vi "My Nonlinear Curve Fit LM bounds.vi"(0 "Y":dbl[](array[numeric]), 1 "f(x,a)":T5, 2 "data":variant, 5 "X":dbl[](array[numeric]), 7 "Weight":dbl[](array[numeric]), 9 "initial parameters":dbl[](array[numeric]), 11 "error in (no error)":errorcluster, 12 "Termination Criteria":T6={"Max Iterations"=1000, "Max Function Calls"=10000, "Max Time"=1000.0, "Function Tolerance"=1e-06, "Parameter Tolerance"=1e-06, "Gradient Tolerance"=1e-06, "Min Lambda"=1e-06, "Max Lambda"=1000000.0, "Initial Tick Count"=0}, 13 "parameter bounds":T3, 14 "NL Fit Method":T4) -> (3 "Fit Aborted?":bool, 4 "best nonlinear fit":dbl[](array[numeric]), 6 "best fit parameters":dbl[](array[numeric]), 8 "covariance":T7, 10 "Fit Statistics":T1={"# Iterations"=0, "# Function Calls"=0, "Chi2"=0.0, "Chi2/DOF"=0.0, "Fit Convergence Criterion"=enum."Continue", "Gradient"=0.0, "|Delta Chi 2|"=0.0, "|Delta Chi 2|/Chi 2"=0.0, "Max |Delta a| /|a|"=0.0, "Lambda"=-1.0, "Weighted Chi2"=-1.0, "Unweighted Chi2"=-1.0}, 15 "error out":errorcluster)   [LabVIEW 2021, in "Fits.lvlib"]
uses:
  Fits.lvlib
  <vilib>/Analysis/Matrix/Datatypes/RealMatrix.ctl
  My Fit Stopping Criteria.ctl
  <vilib>/gmath/NumericalOptimization/LM model function reference.ctl
  Nonlinear Fit Method.ctl
  Fit Statistics v3.ctl
  Convergence Criteria.ctl
  <vilib>/gmath/NumericalOptimization/LM model function.ctl
  <userlib>/_OpenG.lib/array/array.llb/Remove Duplicates from 1D Array (DBL)__ogtk.vi
  Abort Fit Global.vi
  <vilib>/Analysis/baseanly.llb/Real Inverse Matrix.vi
  <vilib>/gmath/NumericalOptimization/LM_output select.ctl
  <vilib>/gmath/NI_Gmath.lvlib
  <vilib>/Analysis/NI_AALBase.lvlib
  <userlib>/_OpenG.lib/array/array.llb/openg_array.lvlib
  <vilib>/Analysis/Matrix/NI_Matrix.lvlib
panel:
  out "Lambda Chart":dbl(graph)
  out "Parameters Gradient Chart":dbl[][](graph)
  in  "Repeat Fit N times (1)":i32=1
  in  "Reset Charts":bool
  out "Chi2 Chart":dbl(graph)
  out "Parameters Graph":dbl[](graph)
  in  "Delay (ms)":i32
  in  "Debug":bool
  out "Parameters Chart":dbl[][](graph)
  out "Function & Fit Graph":cluster{"New Coefficients":dbl[]}[](graph)
  # "see the AlliGator License on the block diagram (Ctrl+E or Window:Show Block Diagram)"
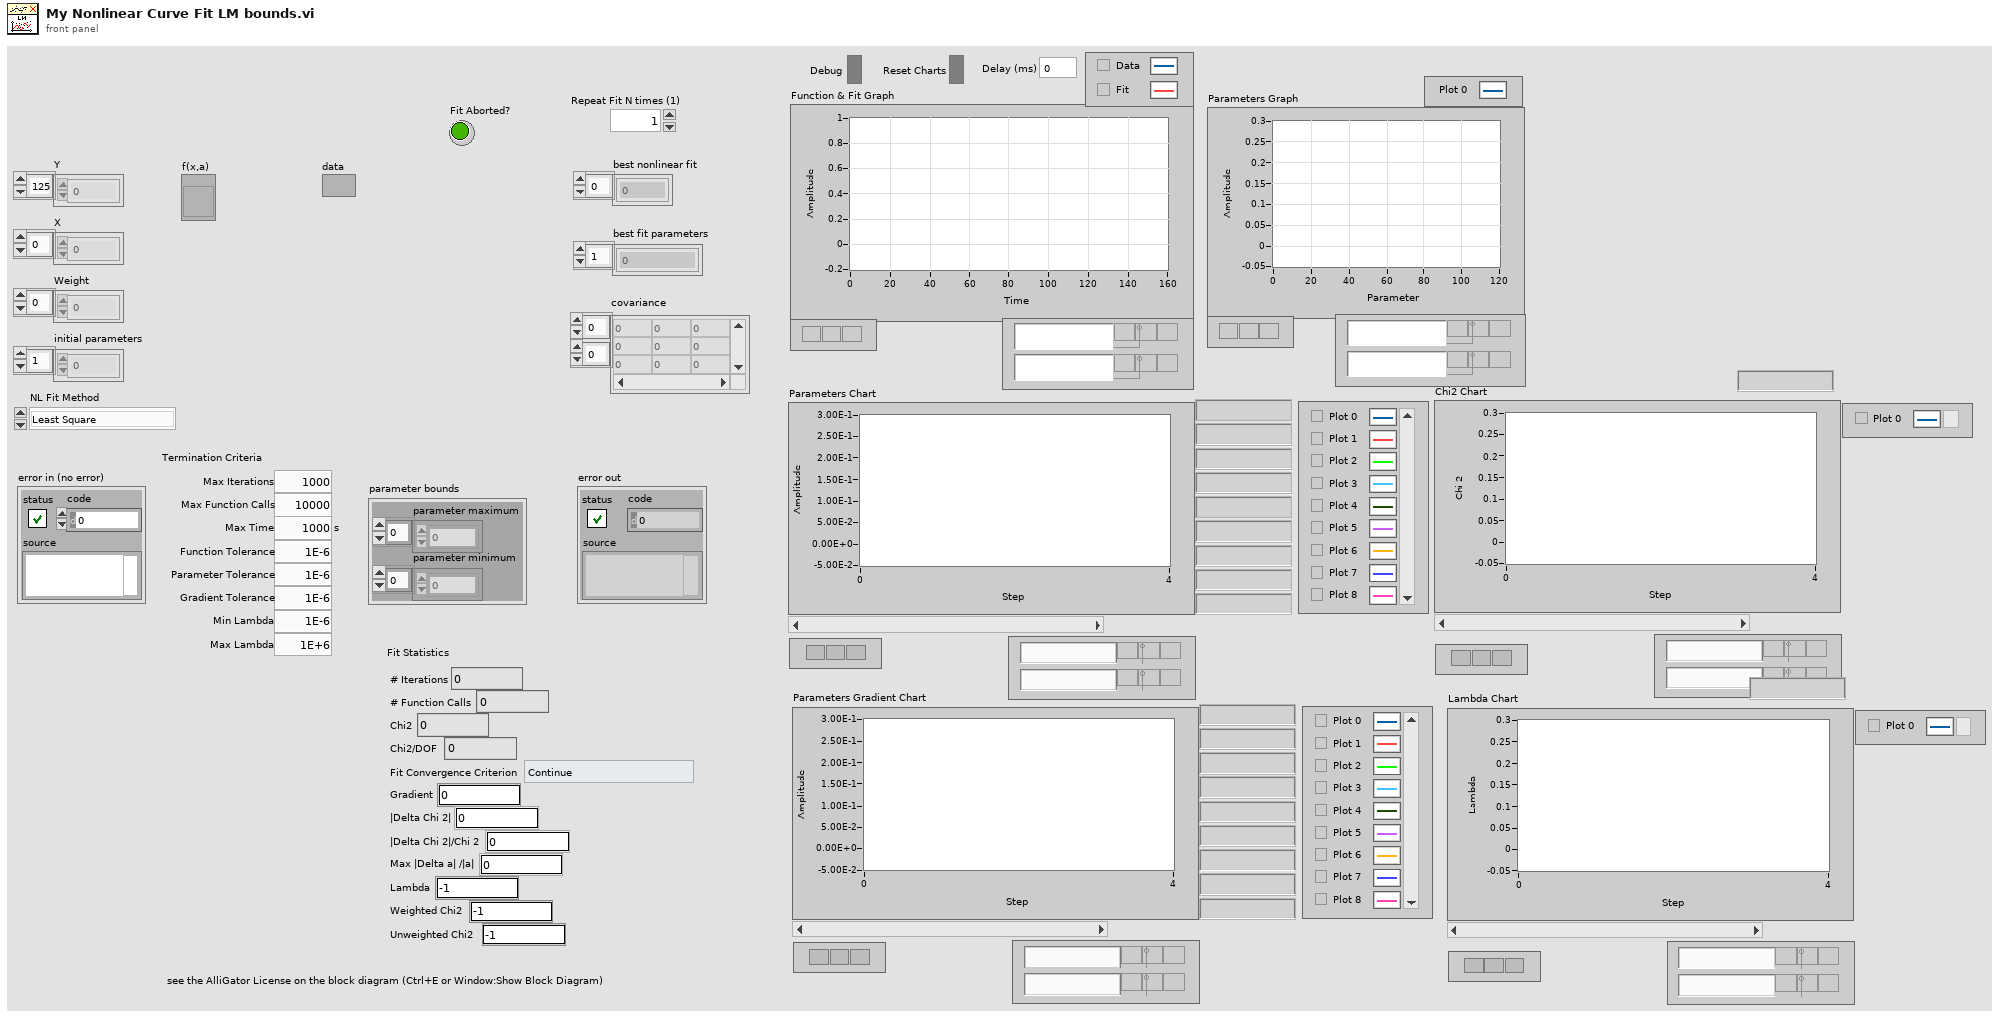
[diagram p1: front panel]
types:
  T1 = typedef "Fits.lvlib/Fit Statistics v3.ctl" = cluster{"# Iterations":i32, "# Function Calls":i32, "Chi2":dbl, "Chi2/DOF":dbl, "Fit Convergence Criterion":T2, "Gradient":dbl, "|Delta Chi 2|":dbl, "|Delta Chi 2|/Chi 2":dbl, "Max |Delta a| /|a|":dbl, "Lambda":dbl, "Weighted Chi2":dbl, "Unweighted Chi2":dbl}
  T2 = typedef "Fits.lvlib/Convergence Criteria.ctl" = enum16{"Continue", "Tolerances Exceeded", "Max Time Exceeded", "Max Iterations Exceeded", "Max Function Evaluations Exceeded", "Scale Range Exceeded"}
  T3 = cluster{"parameter minimum":dbl[], "parameter maximum":dbl[]}
  T4 = typedef "Fits.lvlib/Nonlinear Fit Method.ctl" = enum16{"Least Square", "Least Absolute Residual", "Bisquare", "MLE"}
  T5 = typedef "NI_Gmath.lvlib/LM model function reference.ctl" = refnum<vi>
  T6 = typedef "Fits.lvlib/My Fit Stopping Criteria.ctl" = cluster{"Max Iterations":i32, "Max Function Calls":i32, "Max Time":dbl[unit], "Function Tolerance":dbl, "Parameter Tolerance":dbl, "Gradient Tolerance":dbl, "Min Lambda":dbl, "Max Lambda":dbl, "Initial Tick Count":u32}
  T7 = typedef "NI_Matrix.lvlib/RealMatrix.ctl" = dbl[][]
  T8 = typedef "NI_Gmath.lvlib/LM model function.ctl" = cluster{"f(x,a)":T5, "data":variant}
  T9 = typedef "NI_Gmath.lvlib/LM_output select.ctl" = cluster{"model function":bool, "gradient":bool}
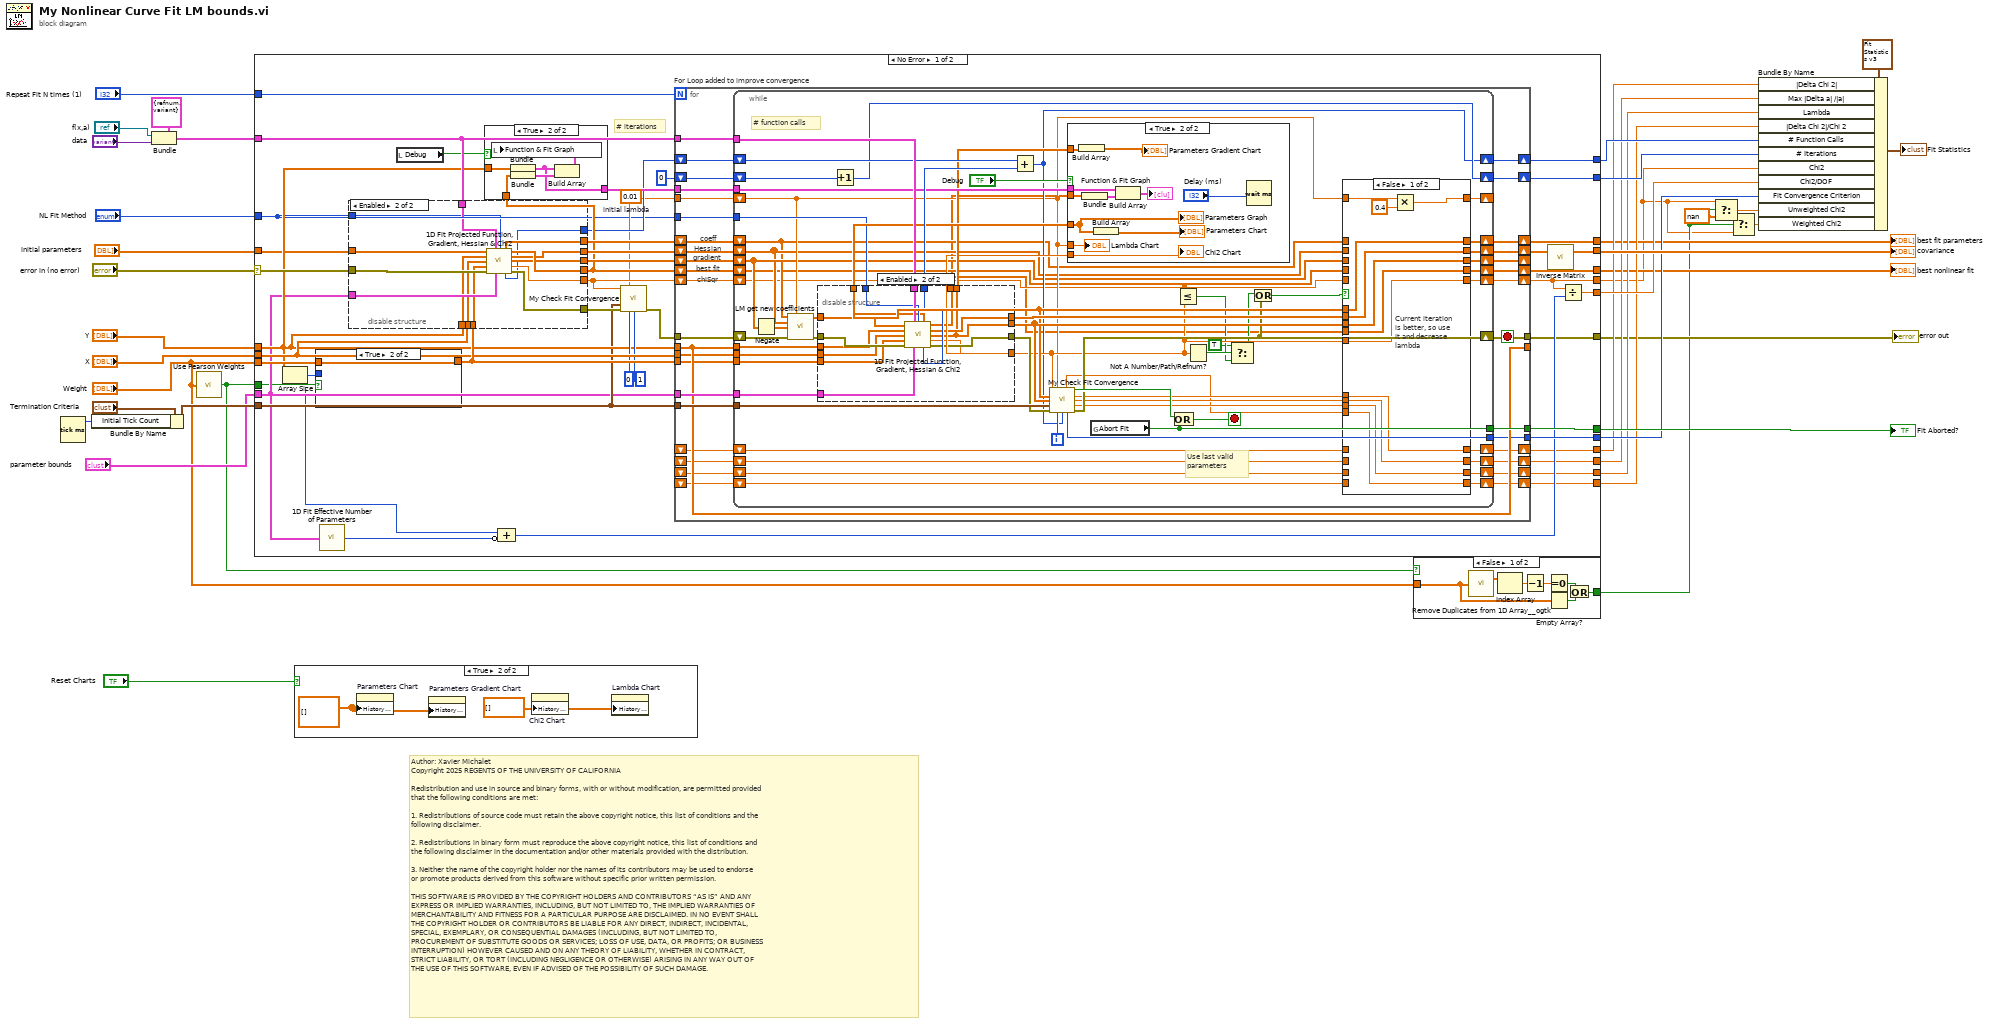
[diagram p0: block diagram]
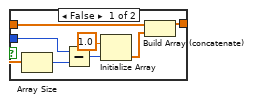
[diagram p3: hidden frame]
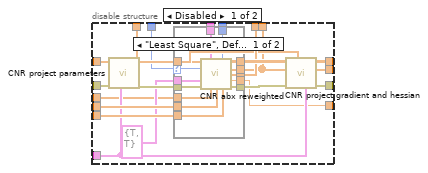
[diagram p4: hidden frame]
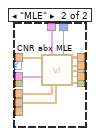
[diagram p5: hidden frame]
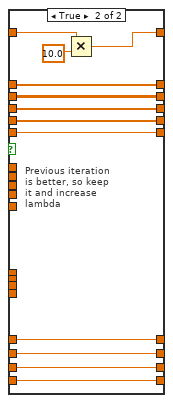
[diagram p7: hidden frame]
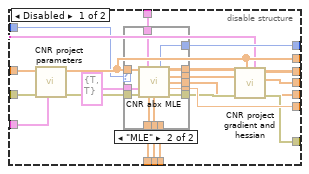
[diagram p8: hidden frame]
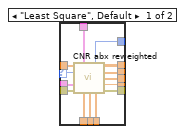
[diagram p9: hidden frame]
diagram:
  w9 = nan ("f")
  # "Author: Xavier Michalet\nCopyright 2025 REGENTS OF THE UNIVERSITY OF CALIFORNIA\n\nRedistribution and use in source and binary forms, with or without modification, are permitted provided\nthat the following conditions are met:\n\n1. Redistributions of source code must retain the above copyright notice, this list of conditions and the\nfollowing disclaimer.\n\n2. Redistributions in binary form must reproduce the above copyright notice, this list of conditions and\nthe following disclaimer in the documentation and/or other materials provided with the distribution.\n\n3. Neither the name of the copyright holder nor the names of its contributors may be used to endorse \nor promote products derived from this software without specific prior written permission.\n\nTHIS SOFTWARE IS PROVIDED BY THE COPYRIGHT HOLDERS AND CONTRIBUTORS “AS IS” AND ANY \nEXPRESS OR IMPLIED WARRANTIES, INCLUDING, BUT NOT LIMITED TO, THE IMPLIED WARRANTIES OF\nMERCHANTABILITY AND FITNESS FOR A PARTICULAR PURPOSE ARE DISCLAIMED. IN NO EVENT SHALL\nTHE COPYRIGHT HOLDER OR CONTRIBUTORS BE LIABLE FOR ANY DIRECT, INDIRECT, INCIDENTAL, \nSPECIAL, EXEMPLARY, OR CONSEQUENTIAL DAMAGES (INCLUDING, BUT NOT LIMITED TO, \nPROCUREMENT OF SUBSTITUTE GOODS OR SERVICES; LOSS OF USE, DATA, OR PROFITS; OR BUSINESS\nINTERRUPTION) HOWEVER CAUSED AND ON ANY THEORY OF LIABILITY, WHETHER IN CONTRACT, \nSTRICT LIABILITY, OR TORT (INCLUDING NEGLIGENCE OR OTHERWISE) ARISING IN ANY WAY OUT OF\nTHE USE OF THIS SOFTWARE, EVEN IF ADVISED OF THE POSSIBILITY OF SUCH DAMAGE."
  n1 = Tick Count (ms)() -> (millisecond timer value=w25:u32)
  n2 = Bundle By Name(cluster="Termination Criteria", "Initial Tick Count"=w25) -> (w24:T6)
  n3 = Bundle(cluster=T8 {"f(x,a)"=refnum, "data"=variant} ("model function"), "f(x,a)"="f(x,a)", "data"="data") -> (w15:T8)
  n4 = call "Use Pearson Weights.vi"("Weight"="Weight") -> ("Use Pearson Weight"=w1:bool)
  n5 = case shown="No Error" "error in (no error)" {
    selector: "error in (no error)" -> [w66 w346]
    tunnel: [w67 _] -> w13
    tunnel: [w80 _] -> w27
    tunnel: "initial parameters" -> [w48 _]
    tunnel: [w73 _] -> w6
    tunnel: [w79 _] -> w36
    tunnel: "Weight" -> [w78 _]
    tunnel: "Y" -> [w60 _]
    tunnel: w24 -> [w53 _]
    tunnel: "X" -> [w74 _]
    tunnel: [w45 w346] -> w5
    tunnel: w15 -> [w75 _]
    tunnel: [w68 _] -> w30
    tunnel: "NL Fit Method" -> [w44 _]
    tunnel: "parameter bounds" -> [w47 _]
    tunnel: [w61 _] -> w31
    tunnel: [w56 _] -> w3
    tunnel: [w54 _] -> w28
    tunnel: "Repeat Fit N times (1)" -> [w51 _]
    tunnel: [w50 _] -> w20
    tunnel: [w43 _] -> w17
    tunnel: [w42 _] -> w19
    tunnel: [w41 _] -> w18
    tunnel: [w40 _] -> w16
    tunnel: w1 -> [w39 _]
    frame No Error {
      w52 = 0.01  # initial lambda
      # "# iterations"
      n6 = Array Size(array=w60) -> (size(s)=w38:i32)
      n7 = case shown="True" w39 {
        tunnel: [w88 w89] -> w81
        tunnel: w78 -> [w83 w89]
        tunnel: w38 -> [w82 _]
        frame False {
          n8 = Array Size(array=w83) -> (size(s)=w86:i32)
          n9 = Subtract(x=w82, y=w86) -> (x-y=w85:i32)
          n10 = Initialize Array(1.0, w85) -> (w84:dbl[])
          n11 = Build Array (concatenate)(w83, w84) -> (w88:dbl[])
        }
        frame True {
        }
      }
      n12 = call "1D Fit Effective Number of Parameters.vi"("parameter bounds"=w47) -> ("Effective Number of Parameters"=w46:i32)  [unwired: 8 in]
      n13 = disable-structure shown="Enabled" {
        disable-tunnel: w81 -> [w299 w329]
        disable-tunnel: [w298 w337] -> w77
        disable-tunnel: w75 -> [w297 w340]
        disable-tunnel: w74 -> [w296 w328]
        disable-tunnel: w66 -> [w294 w330]
        disable-tunnel: [w291 w336] -> w65
        disable-tunnel: [w288 w339] -> w64
        disable-tunnel: [w287 w335] -> w63
        disable-tunnel: [w286 w334] -> w62
        disable-tunnel: w60 -> [w285 w327]
        disable-tunnel: [w284 w338] -> w58
        disable-tunnel: [w283 w333] -> w55
        disable-tunnel: w48 -> [w282 w326]
        disable-tunnel: w47 -> [w281 w331]
        disable-tunnel: w44 -> [w280 w332]
        frame Disabled {
          n14 = call <vilib>:"CNR project parameters.vi"("bounds"=w281, "error in"=w294, "parameters"=w282) -> ("error out"=w293:errorcluster, "projected parameters"=w288:dbl[])  [unwired: 7 out]
          n15 = case shown="\"MLE\"" w280 {
            selector: w280 -> [w303 _]
            tunnel: w299 -> [w313 _]
            tunnel: [w312 w318] -> w298
            tunnel: w297 -> [w311 w325]
            tunnel: w296 -> [w310 w319]
            tunnel: T9 {"model function"=TRUE, "gradient"=TRUE} ("output control") -> [w309 w323]
            tunnel: w293 -> [w308 w322]
            tunnel: [w307 w321] -> w292
            tunnel: [w306 w315] -> w290
            tunnel: [w305 w316] -> w289
            tunnel: w288 -> [w304 w324]
            tunnel: w285 -> [w302 w320]
            tunnel: [w301 w317] -> w284
            tunnel: [w300 w314] -> w283
            frame "Least Square", Default {
              n16 = call <vilib>:"CNR abx reweighted.vi"("parameters"=w304, "model function"=w311, "method"=w303, "output control"=w309, "error in (no error)"=w308, "Y"=w302, "X"=w310, "Weight"=w313) -> ("number of function calls"=w300:i32, "Hessian"=w306:T7, "gradient"=w305:dbl[], "best fit"=w301:dbl[], "chiSqr"=w312:dbl, "error out"=w307:errorcluster)  [unwired: 1 in, 1 out]
            }
            frame "MLE" {
              n17 = call "CNR abx MLE.vi"("parameters"=w324, "model function"=w325, "output control"=w323, "error in (no error)"=w322, "Y"=w320, "X"=w319) -> ("number of function calls"=w314:i32, "Hessian"=w315:T7, "gradient"=w316:dbl[], "best fit"=w317:dbl[], "chiSqr"=w318:dbl, "error out"=w321:errorcluster)  [unwired: 3 in, 1 out]
            }
          }
          n18 = call <vilib>:"CNR project gradient and hessian.vi"("bounds"=w281, "projected parameters"=w288, "error in"=w292, "gradient"=w289, "Hessian"=w290) -> ("error out"=w291:errorcluster, "projected gradient"=w286:dbl[], "projected Hessian"=w287:T7)  [unwired: 1 in, 3 out]
        }
        frame Enabled {
          n19 = call "1D Fit Projected Function, Gradient, Hessian & Chi2.vi"("parameters"=w326, "model function"=w340, "NL Fit Method"=w332, "Y"=w327, "X"=w328, "Weights"=w329, "Error In"=w330, "Parameter Bounds"=w331) -> ("projected parameters"=w339:dbl[], "best fit"=w338:dbl[], "projected Hessian"=w335:T7, "projected gradient"=w334:dbl[], "Chi2"=w337:dbl, "number of function calls"=w333:i32, "Error Out"=w336:errorcluster)  [unwired: 1 in]
        }
      }
      n20 = local read "Debug"() -> (w57:bool)
      n21 = case shown="True" w57 {
        tunnel: w60 -> [_ w345]
        tunnel: [_ w342] -> w59
        tunnel: w58 -> [_ w344]
        frame False {
        }
        frame True {
          n22 = Bundle("Y"=w345) -> (w342:cluster{"Y":dbl[]})  [unwired: 1 in]
          n23 = Bundle("best fit"=w344) -> (w343:cluster{"best fit":dbl[]})  [unwired: 1 in]
          n24 = Build Array(w342, w343) -> (w341:cluster{"best fit":dbl[]}[])
          n25 = local write "Function & Fit Graph"(w341) -> ()
        }
      }
      n26 = Compound Arithmetic op=ADD(w38, invert w46) -> (w49:i32)
      n27 = call "My Check Fit Convergence.vi"("Chi 2"=w77, "Lambda"=w52, "my stopping criteria"=w53, "Error In"=w65, "current iteration"=0, "number of function evaluations"=1) -> ("error out"=w76:errorcluster)  [unwired: 2 in, 7 out]
      n28 = for "For Loop added to improve convergence" {
        N: w51 -> [_]
        tunnel: w75 -> [w122]
        tunnel: w47 -> [w115]
        tunnel: w44 -> [w112]
        tunnel: [w111] -> w61
        tunnel: w59 -> [w110]
        tunnel: w53 -> [w105]
        shift-right: [w108] -> w56
        shift-left: w77 -> [w124]
        shift-right: [w118] -> w68
        shift-left: w55 -> [w107]
        shift-right: [w106] -> w54
        shift-left: 0 -> [w119]
        tunnel: w52 -> [w104]
        shift-right: [w117] -> w67
        shift-left: w64 -> [w116]
        shift-right: [w120] -> w70
        shift-left: w63 -> [w114]
        shift-right: [w103] -> _
        shift-left: w62 -> [w113]
        shift-right: [w121] -> w73
        shift-left: w58 -> [w109]
        tunnel: [w99] -> w50
        tunnel: w76 -> [w123]
        tunnel: [w98] -> w45
        shift-right: [w96] -> w42
        shift-left: _ -> [w92]
        shift-right: [w97] -> w43
        shift-left: _ -> [w91]
        shift-right: [w95] -> w41
        shift-left: _ -> [w93]
        shift-right: [w94] -> w40
        shift-left: _ -> [w90]
        tunnel: w81 -> [w100]
        tunnel: w74 -> [w101]
        tunnel: w60 -> [w102]
        tunnel: [w102] -> _
        stop <- w98 stop-if-true
        # "best fit"
        # "chiSqr"
        # "gradient"
        # "Hessian"
        # "coeff"
        n29 = while {
          tunnel: w101 -> [w179]
          tunnel: w102 -> [w161]
          tunnel: w100 -> [w178]
          shift-left: w124 -> [w126]
          shift-right: [w170] -> w108
          shift-left: w113 -> [w130]
          shift-right: [w182] -> w103
          shift-left: w114 -> [w129]
          shift-right: [w183] -> w120
          shift-left: w116 -> [w128]
          shift-right: [w171] -> w117
          shift-left: w104 -> [w131]
          shift-right: [w180] -> _
          shift-right: [w152] -> w98
          shift-left: w123 -> [w181]
          tunnel: w122 -> [w177]
          tunnel: w105 -> [w173]
          shift-right: [w132] -> w118
          shift-left: w107 -> [w176]
          shift-right: [w175] -> w121
          shift-left: w109 -> [w127]
          shift-right: [w133] -> w106
          shift-left: w119 -> [w158]
          tunnel: w112 -> [w146]
          tunnel: w115 -> [w166]
          tunnel: [w163] -> w111
          tunnel: w110 -> [w160]
          tunnel: [w154] -> w99
          shift-right: [w141] -> w95
          shift-left: w93 -> [w137]
          shift-right: [w140] -> w96
          shift-left: w92 -> [w136]
          shift-right: [w139] -> w97
          shift-left: w91 -> [w135]
          shift-right: [w138] -> w94
          shift-left: w90 -> [w134]
          i -> [w157]
          stop <- w156 stop-if-true
          # "# function calls"
          # "Use last valid parameters"
          n30 = Negate(x=w130) -> (-x=w164:dbl[])
          n31 = call <vilib>:"LM get new coefficients.vi"("Coefficients"=w128, "lamda"=w131, "Alpha"=w129, "Beta"=w164, "error in (no error)"=w181) -> ("New Coefficients"=w162:dbl[], "error out"=w169:errorcluster)  [unwired: 9 out]
          n32 = disable-structure shown="Enabled" {
            disable-tunnel: [w204 w243] -> w184
            disable-tunnel: w179 -> [w203 w231]
            disable-tunnel: w178 -> [w202 w230]
            disable-tunnel: w177 -> [w201 w244]
            disable-tunnel: w169 -> [w200 w241]
            disable-tunnel: [w197 w242] -> w168
            disable-tunnel: [w196 w235] -> w167
            disable-tunnel: w166 -> [w195 w240]
            disable-tunnel: [w193 w237] -> w165
            disable-tunnel: w162 -> [w191 w239]
            disable-tunnel: w161 -> [w190 w232]
            disable-tunnel: [w189 w236] -> w125
            disable-tunnel: [w188 w233] -> w155
            disable-tunnel: [w187 w235] -> w153
            disable-tunnel: [w186 w238] -> w151
            disable-tunnel: w146 -> [w185 w234]
            frame Disabled {
              n33 = call <vilib>:"CNR project parameters.vi"("bounds"=w195, "error in"=w200, "parameters"=w191) -> ("error out"=w199:errorcluster, "projected parameters"=w188:dbl[])  [unwired: 7 out]
              n34 = case shown="\"Least Square\", Default" w185 {
                selector: w185 -> [w210 _]
                tunnel: [w218 w224] -> w204
                tunnel: w203 -> [w217 w225]
                tunnel: w202 -> [w216 _]
                tunnel: w201 -> [w215 w228]
                tunnel: w199 -> [w214 _]
                tunnel: [w213 w219] -> w198
                tunnel: [w212 w223] -> w194
                tunnel: T9 {"model function"=TRUE, "gradient"=TRUE} ("output control") -> [w211 w227]
                tunnel: w190 -> [w209 w226]
                tunnel: [w208 w221] -> w189
                tunnel: w188 -> [w207 w229]
                tunnel: [w206 w222] -> w187
                tunnel: [w205 w220] -> w186
                frame "Least Square", Default {
                  n35 = call <vilib>:"CNR abx reweighted.vi"("parameters"=w207, "model function"=w215, "method"=w210, "output control"=w211, "error in (no error)"=w214, "Y"=w209, "X"=w217, "Weight"=w216) -> ("number of function calls"=w218:i32, "Hessian"=w212:T7, "gradient"=w206:dbl[], "best fit"=w208:dbl[], "chiSqr"=w205:dbl, "error out"=w213:errorcluster)  [unwired: 1 in, 1 out]
                }
                frame "MLE" {
                  n36 = call "CNR abx MLE.vi"("parameters"=w229, "model function"=w228, "output control"=w227, "Y"=w226, "X"=w225) -> ("number of function calls"=w224:i32, "Hessian"=w223:T7, "gradient"=w222:dbl[], "best fit"=w221:dbl[], "chiSqr"=w220:dbl, "error out"=w219:errorcluster)  [unwired: 4 in, 1 out]
                }
              }
              n37 = call <vilib>:"CNR project gradient and hessian.vi"("bounds"=w195, "projected parameters"=w188, "error in"=w198, "gradient"=w187, "Hessian"=w194) -> ("error out"=w197:errorcluster, "projected gradient"=w196:dbl[], "projected Hessian"=w193:T7)  [unwired: 1 in, 3 out]
            }
            frame Enabled {
              n38 = call "1D Fit Projected Function, Gradient, Hessian & Chi2.vi"("parameters"=w239, "model function"=w244, "NL Fit Method"=w234, "Y"=w232, "X"=w231, "Weights"=w230, "Error In"=w241, "Parameter Bounds"=w240) -> ("projected parameters"=w233:dbl[], "best fit"=w236:dbl[], "projected Hessian"=w237:T7, "projected gradient"=w235:dbl[], "Chi2"=w238:dbl, "number of function calls"=w243:i32, "Error Out"=w242:errorcluster)  [unwired: 1 in]
            }
          }
          n39 = Increment(x=w158) -> (x+1=w133:i32)
          n40 = Add(x=w176, y=w184) -> (x+y=w132:i32)
          n41 = call "My Check Fit Convergence.vi"("Chi 2"=w151, "Lambda"=w131, "Parameters"=w155, "gradient"=w167, "my stopping criteria"=w173, "Error In"=w168, "current iteration"=w157, "number of function evaluations"=w132) -> ("|Delta Chi 2|/Chi 2"=w142:dbl, "stop?"=w172:bool, "|Delta Chi 2|"=w145:dbl, "Max |Delta a| /|a|"=w144:dbl, "Lambda"=w143:dbl, "Convergence Criterium Reached"=w154:T2, "error out"=w152:errorcluster)  [unwired: 1 out]
          n42 = case shown="True" "Debug" {
            tunnel: w155 -> [_ w248]
            tunnel: w160 -> [_ w255]
            tunnel: w125 -> [_ w252]
            tunnel: w151 -> [_ w250]
            tunnel: w153 -> [_ w249]
            tunnel: w131 -> [_ w245]
            frame False {
            }
            frame True {
              n43 = Build Array(w249) -> (→"Parameters Gradient Chart":dbl[][])
              n44 = Bundle("best fit"=w252) -> (w254:cluster{"best fit":dbl[]})  [unwired: 1 in]
              n45 = Build Array(w248) -> (→"Parameters Chart":dbl[][])
              n46 = Build Array(w255, w254) -> (→"Function & Fit Graph":cluster{"best fit":dbl[]}[])
              n47 = Wait (ms)(milliseconds to wait="Delay (ms)") -> ()  [unwired: 1 out]
              "Parameters Graph" <- w248
              "Chi2 Chart" <- w250
              "Lambda Chart" <- w245
            }
          }
          n48 = global read "Abort Fit Global.vi" "Abort Fit"() -> (w163:bool)
          n49 = Compound Arithmetic op=OR(w172, w163) -> (w156:bool)
          n50 = Less Or Equal?(x=w126, y=w151) -> (x <= y?=w149:bool)
          n51 = Not A Number/Path/Refnum?(number/path/refnum=w151) -> (NaN/Path/Refnum?=w150:bool)
          n52 = Select(t=TRUE, s=w150, f=w149) -> (s? t:f=w147:bool)
          n53 = Or(x=w147, y=w152) -> (x .or. y?=w174:bool)
          n54 = case shown="False" w174 {
            tunnel: [w266 w279] -> w183
            tunnel: w129 -> [_ w279]
            tunnel: [w265 w278] -> w182
            tunnel: w155 -> [w262 _]
            tunnel: w130 -> [_ w278]
            tunnel: w128 -> [_ w277]
            tunnel: [w262 w277] -> w171
            tunnel: [w267 w275] -> w180
            tunnel: w126 -> [_ w276]
            tunnel: w151 -> [w263 _]
            tunnel: [w263 w276] -> w170
            tunnel: w131 -> [w261 w273]
            tunnel: w165 -> [w266 _]
            tunnel: w167 -> [w265 _]
            tunnel: w127 -> [_ w274]
            tunnel: w125 -> [w264 _]
            tunnel: [w264 w274] -> w175
            tunnel: w145 -> [w259 _]
            tunnel: w144 -> [w258 _]
            tunnel: w143 -> [w257 _]
            tunnel: w142 -> [w256 _]
            tunnel: [w259 w271] -> w141
            tunnel: [w258 w270] -> w140
            tunnel: [w257 w269] -> w139
            tunnel: [w256 w268] -> w138
            tunnel: w137 -> [_ w271]
            tunnel: w136 -> [_ w270]
            tunnel: w135 -> [_ w269]
            tunnel: w134 -> [_ w268]
            frame False {
              # "Current iteration\nis better, so use\nit and decrease \nlambda"
              n55 = Multiply(x=w261, y=0.4) -> (x*y=w267:dbl)
            }
            frame True {
              # "Previous iteration\nis better, so keep\nit and increase \nlambda"
              n56 = Multiply(x=w273, y=10.0) -> (x*y=w275:dbl)
            }
          }
        }
      }
      n57 = call-poly <vilib>:"Inverse Matrix.vi"("Input Matrix"=w70) -> ("Inverse Matrix"=w79:T7)  [unwired: 1 in, 1 out]
      n58 = Divide(x=w56, y=w49) -> (x/y=w80:dbl)
    }
    frame Error {
    }
  }
  "best fit parameters" <- w13
  "best nonlinear fit" <- w6
  "error out" <- w5
  "covariance" <- w36
  "Fit Aborted?" <- w31
  n59 = case shown="True" "Reset Charts" {
    frame False {
    }
    frame True {
      w347 = dbl[] [] ("History Data")
      w348 = dbl[][] [] ("History Data")
      n60 = property on="Parameters Chart" class="WFChart (strict)"("History Data"=w348) -> ()  [unwired: 2 in, 2 out]
      n61 = property on="Parameters Gradient Chart" class="WFChart (strict)"("History Data"=w348) -> ()  [unwired: 2 in, 2 out]
      n62 = property on="Chi2 Chart" class="WFChart (strict)"("History Data"=w347) -> ()  [unwired: 2 in, 2 out]
      n63 = property on="Lambda Chart" class="WFChart (strict)"("History Data"=w347) -> ()  [unwired: 2 in, 2 out]
    }
  }
  n64 = case shown="False" w1 {
    tunnel: [w350 _] -> w4
    tunnel: "Weight" -> [w349 _]
    frame False {
      n65 = call-poly <userlib>:"Remove Duplicates from 1D Array__ogtk.vi"("Input Array"=w349) -> ("Output Array"=w352:dbl[])  [unwired: 1 out]
      n66 = Index Array(array=w352) -> (element=w351:dbl)  [unwired: 1 in]
      n67 = Decrement(x=w351) -> (x-1=w355:dbl)
      n68 = Equal To 0?(x=w355) -> (x = 0?=w354:bool)
      n69 = Empty Array?(array=w349) -> (empty?=w353:bool)
      n70 = Or(x=w354, y=w353) -> (x .or. y?=w350:bool)
    }
    frame True {
    }
  }
  n71 = Select(t=w3, s=w4, f=w9) -> (s? t:f=w10:dbl)
  n72 = Select(t=w9, s=w4, f=w3) -> (s? t:f=w8:dbl)
  n73 = Bundle By Name(cluster=T1 {"# Iterations"=0, "# Function Calls"=0, "Chi2"=0.0, "Chi2/DOF"=0.0, "Fit Convergence Criterion"=enum."Continue", "Gradient"=0.0, "|Delta Chi 2|"=0.0, "|Delta Chi 2|/Chi 2"=0.0, "Max |Delta a| /|a|"=0.0, "Lambda"=-1.0, "Weighted Chi2"=-1.0, "Unweighted Chi2"=-1.0} ("Fit Statistics"), "|Delta Chi 2|"=w18, "Max |Delta a| /|a|"=w19, "Lambda"=w17, "|Delta Chi 2|/Chi 2"=w16, "# Function Calls"=w30, "# Iterations"=w28, "Chi2"=w3, "Chi2/DOF"=w27, "Fit Convergence Criterion"=w20, "Unweighted Chi2"=w10, "Weighted Chi2"=w8) -> (→"Fit Statistics":T1)
